vi "Set Ring Light.vi"(8 "error in":errorcluster, 11 "Light On? (F)":bool) -> (0 "error out":errorcluster)   [LabVIEW 2016, in "Vision Drive.lvlib"]
uses:
  Vision Drive.lvlib
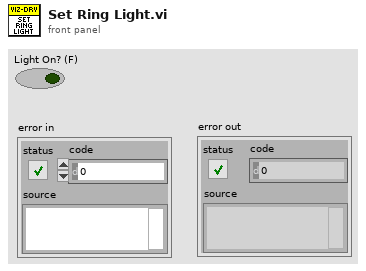
[diagram p1: front panel]
types:
  T1 = typedef "WPI_DigitalOutputDevRef.ctl" = cluster{"DIO Channel":T2, "DevStatus":errorcluster}
  T2 = typedef "FPGA_DIOChannel.ctl" = enum8{"DIO 0", "DIO 1", "DIO 2", "DIO 3", "DIO 4", "DIO 5", "DIO 6", "DIO 7", "DIO 8", "DIO 9", "DIO MXP 0", "DIO MXP 1", "DIO MXP 2", "DIO MXP 3", "DIO MXP 4", "DIO MXP 5", "DIO MXP 6", "DIO MXP 7", "DIO MXP 8", "DIO MXP 9", "DIO MXP 10", "DIO MXP 11", "DIO MXP 12", "DIO MXP 13", "DIO MXP 14", "DIO MXP 15", "SPI Port CS1", "SPI Port CS2", "SPI Port CS3", "SPI Port MISO", "SPI Port MOSI", "Invalid"}
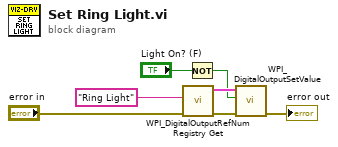
[diagram p0: block diagram]
diagram:
  n1 = call <vilib>:"WPI_DigitalOutputRefNum Registry Get.vi"("error in (no error)"="error in", "refnum name"="Ring Light") -> ("error out"=w6:errorcluster, "DigitalOutputDevRef"=w3:T1)  [unwired: 8 in]
  n2 = Not(x="Light On? (F)") -> (.not. x?=w1:bool)
  n3 = call <vilib>:"WPI_DigitalOutputSetValue.vi"("error in (no error)"=w6, "Value"=w1, "DigitalOutputDevRef"=w3) -> ("error out"=→"error out":errorcluster)  [unwired: 7 in, 1 out]
